vi "Set Site Relay Driver And Relay Supply.vi"(0 "TSM Context":T1, 5 "DAQmx Task":refnum<k21>, 7 "SSC.Channels":string, 9 "State (F:Enable)":bool, 11 "error in":errorcluster) -> (15 "error out":errorcluster)   [LabVIEW 2019]
uses:
  <vilib>/NI_TestStand_SemiconductorModule/NI_TestStand_Semiconductor_Module.lvlibp/PinMap/General/SemiconductorModuleContext.ctl
  TSM Context Data Access/TSM Context Data Access.lvclass/TSM Context Data Access.ctl
  <vilib>/DAQmx/write.llb/DAQmx Write (Digital 1D Bool 1Chan 1Samp).vi
  TSM Context Data Access/Public/Properties/DAQ Port1 State - Read.vi
  TSM Context Data Access/Public/Properties/DAQ Port1 State - Write.vi
  <vilib>/NI_TestStand_SemiconductorModule/NI_TestStand_Semiconductor_Module.lvlibp/PinMap/Site and Global Data/GetGlobalData.vi
  TSM Context Data Access/Public/Properties/DAQ Port1 Pins - Read.vi
  <vilib>/NI_TestStand_SemiconductorModule/NI_TestStand_Semiconductor_Module.lvlibp/PinMap/Site and Global Data/SetGlobalData.vi
  <vilib>/DAQmx/miscellaneous.llb/DAQmx Fill In Error Info.vi
  <vilib>/NI_TestStand_SemiconductorModule/NI_TestStand_Semiconductor_Module.lvlibp
  TSM Context Data Access/TSM Context Data Access.lvclass
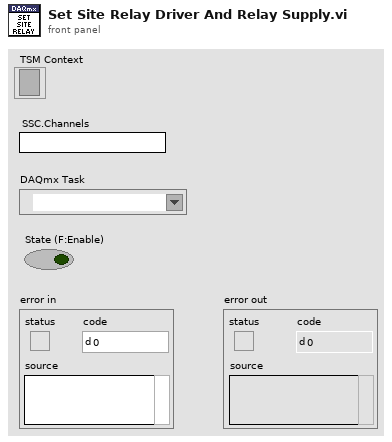
[diagram p1: front panel]
types:
  T1 = typedef "NI_TestStand_Semiconductor_Module.lvlibp/SemiconductorModuleContext.ctl" = refnum<k7>
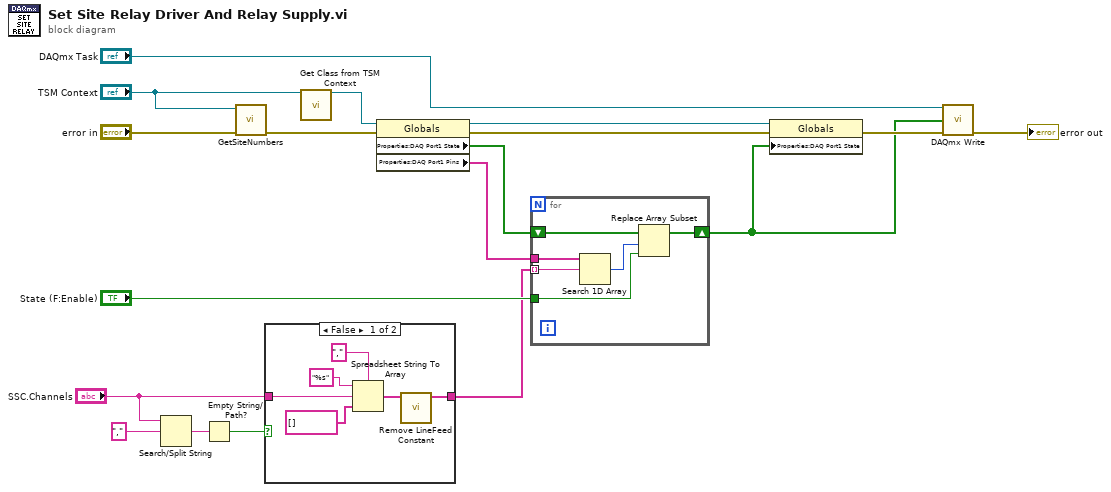
[diagram p0: block diagram]
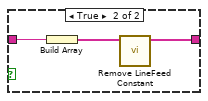
[diagram p2: hidden frame]
diagram:
  n1 = Search/Split String(string="SSC.Channels", search string/char (-)=",") -> (match + rest of string=w5:string)  [unwired: 1 in, 2 out]
  n2 = Empty String/Path?(string/path=w5) -> (empty?=w4:bool)
  n3 = call <vilib>:"GetSiteNumbers.vi"("error in (no error)"="error in", "Semiconductor Module Context"="TSM Context") -> ("error out"=w15:errorcluster)  [unwired: 6 in, 3 out]
  n4 = case shown="False" w4 {
    tunnel: "SSC.Channels" -> [w24 w27]
    tunnel: [w19 w25] -> w1
    frame False {
      n5 = Spreadsheet String To Array(delimiter (Tab)=",", format string="%s", spreadsheet string=w24, array type (2D Dbl)=string[] [] ("format string")) -> (array=w20:string[])
      n6 = call "Remove LineFeed Constant.vi"("1D String Array in"=w20) -> ("1D String Array out"=w19:string[])  [unwired: 10 in]
    }
    frame True {
      n7 = Build Array(w27) -> (w26:string[])
      n8 = call "Remove LineFeed Constant.vi"("1D String Array in"=w26) -> ("1D String Array out"=w25:string[])  [unwired: 10 in]
    }
  }
  n9 = call "Get Class from TSM Context.vi"("TSM Context"="TSM Context") -> ("Global Memory Class"=w11:refnum<class "TSM Context Data Access.lvclass">)  [unwired: 14 in]
  n10 = property class="Globals"(reference=w11, error in=w15) -> (reference out=w8:refnum<class "TSM Context Data Access.lvclass">, error out=w13:errorcluster, "Properties:DAQ Port1 State"=w10:bool[], "Properties:DAQ Port1 Pins"=w2:string[])
  n11 = for {
    tunnel: "State (F:Enable)" -> [w30]
    shift-right: [w32] -> w7
    shift-left: w10 -> [w33]
    tunnel: w2 -> [w29]
    tunnel: w1 -> [w28] mode=indexing
    n12 = Search 1D Array(1D array=w29, element=w28) -> (index of element=w31:i32)  [unwired: 1 in]
    n13 = Replace Array Subset(array=w33, new element=w30, index=w31) -> (w32:bool[])
  }
  n14 = property class="Globals"(reference=w8, error in=w13, "Properties:DAQ Port1 State"=w7) -> (error out=w9:errorcluster)  [unwired: 1 out]
  n15 = call-poly <vilib>:"DAQmx Write.vi"("task/channels in"="DAQmx Task", "data"=w7, "error in"=w9) -> ("error out"=→"error out":errorcluster)  [unwired: 10 in, 2 out]
